vi "Stack_holderwise_total_bd_count_&_duration_3_for_stationwise.vi"(0 "Refnum in":T1, 1 "BREAKDOWN_STK_HOLD_ID":i32=1, 2 "condition":string="Where BREAKDOWN_DATE between '%s'and '%s' and BREAKDOWN_STK_HOLD_ID ='%d'  ", 5 "Form Date":timestamp, 7 "Array":string[](array[string]), 9 "To Date":timestamp, 11 "error in (no error)":errorcluster, 12 "STATION_ID_CID_TRIGGER":i32, 13 "Shift":string(combo), 14 "table":string[](array[string])=["STATION_1_LOG_HISTORY"]) -> (4 "Refnum out":T1, 6 "Count out":string[](array[string]), 10 "appended array":dbl[](array[numeric]), 15 "error out":errorcluster)   [LabVIEW 2017]
uses:
  <vilib>/addons/database/Connection.llb/Conn ObjectReference.ctl
  <vilib>/addons/database/NI_Database_API.lvlib
panel:
  out "Count out 2":string[](array[string])
  out "Table":string[][](array[string])
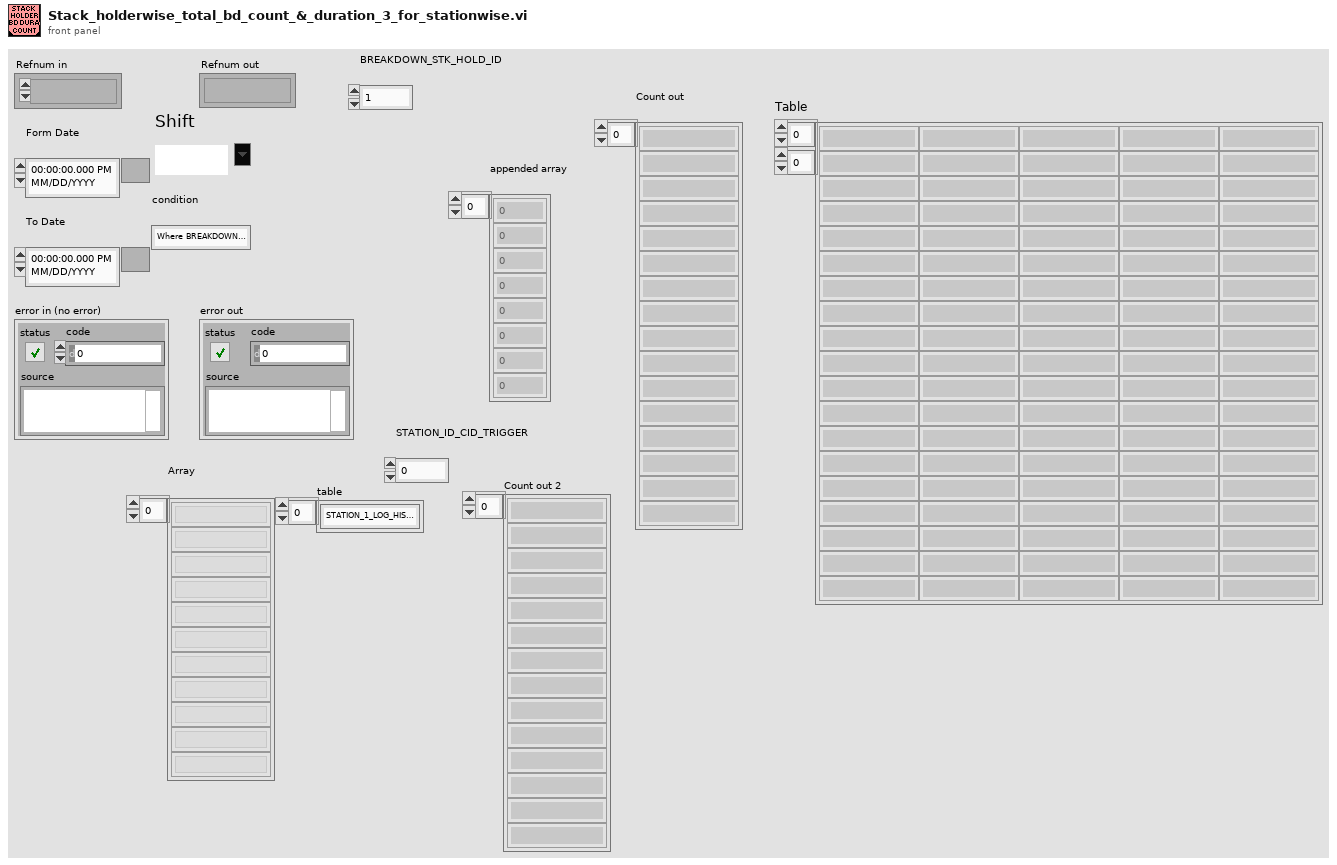
[diagram p1: front panel]
types:
  T1 = typedef "NI_Database_API.lvlib/Conn ObjectReference.ctl" = refnum<k1>
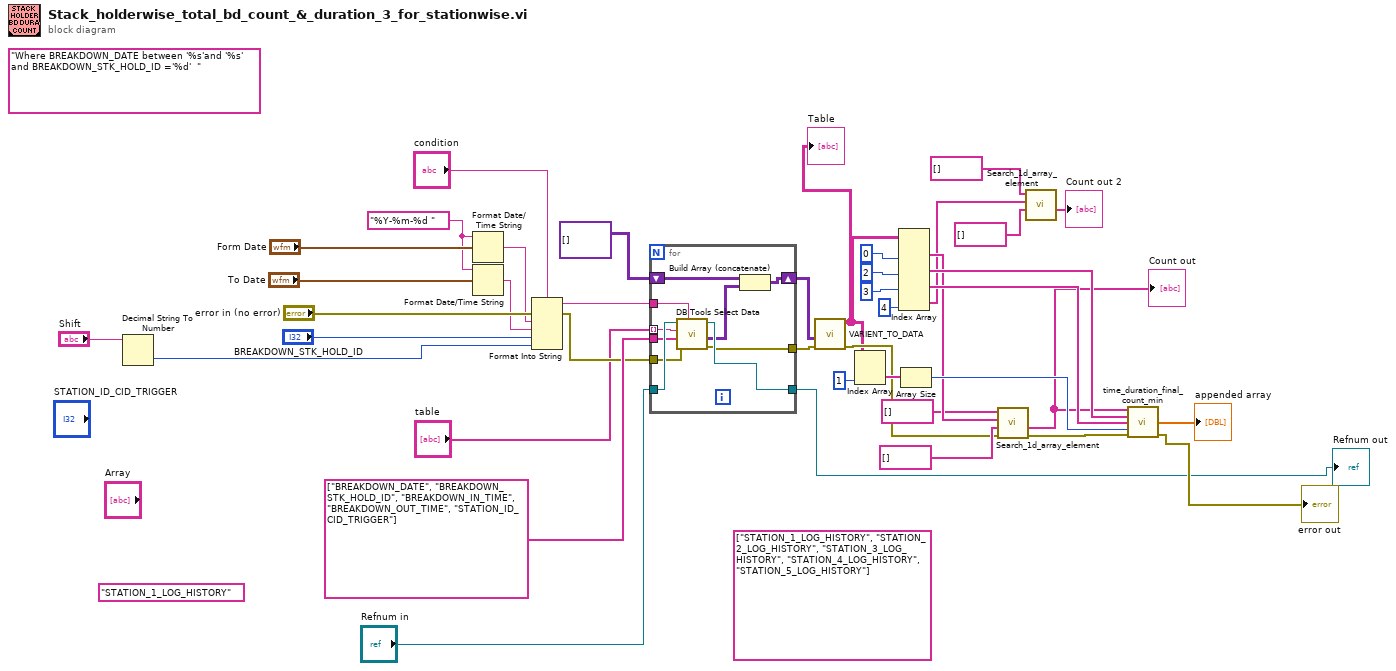
[diagram p0: block diagram]
diagram:
  (unwired) string[] ["STATION_1_LOG_HISTORY", "STATION_2_LOG_HISTORY", "STATION_3_LOG_HISTORY", "STATION_4_LOG_HISTORY", "STATION_5_LOG_HISTORY"]
  (unwired) "Where BREAKDOWN_DATE between '%s'and '%s' and BREAKDOWN_STK_HOLD_ID ='%d'  "
  (unwired) "STATION_1_LOG_HISTORY" ("table")
  w19 = "%Y-%m-%d " ("time format string (%c)")
  n1 = Decimal String To Number(string="Shift") -> (number=w12:i32)  [unwired: 2 in, 1 out]
  n2 = Format Date/Time String(time format string (%c)=w19, seconds (now)="Form Date") -> (date/time string=w22:string)  [unwired: 1 in]
  n3 = Format Date/Time String(time format string (%c)=w19, seconds (now)="To Date") -> (date/time string=w23:string)  [unwired: 1 in]
  n4 = Format Into String(format string="condition", error in="error in (no error)", w22, w23, "BREAKDOWN_STK_HOLD_ID", w12) -> (resulting string=w17:string, error out=w18:errorcluster)  [unwired: 1 in]
  n5 = for {
    tunnel: string[] ["BREAKDOWN_DATE", "BREAKDOWN_STK_HOLD_ID", "BREAKDOWN_IN_TIME", "BREAKDOWN_OUT_TIME", "STATION_ID_CID_TRIGGER"] -> [w47]
    tunnel: w17 -> [w48]
    tunnel: w18 -> [w49]
    tunnel: "table" -> [w46] mode=indexing
    tunnel: "Refnum in" -> [w50]
    tunnel: [w51] -> w26
    shift-right: [w44] -> w2
    shift-left: variant[][] [] ("data") -> [w45]
    tunnel: [w42] -> w4
    n6 = call <vilib>:"DB Tools Select Data.vi"("condition"=w48, "error in (no error)"=w49, "columns"=w47, "table"=w46, "connection reference"=w50) -> ("error out"=w42:errorcluster, "data"=w43:variant[][], "connection reference out"=w51:T1)  [unwired: 1 in]
    n7 = Build Array (concatenate)(w45, w43) -> (w44:variant[][])
  }
  "Refnum out" <- w26
  n8 = call "VARIENT_TO_DATA.vi"("data"=w2, "error in (no error)"=w4) -> ("Table"=w1:string[][], "error out"=w3:errorcluster)  [unwired: 7 in]
  "Table" <- w1
  n9 = Index Array(array=w1, index (col)=1 ("disabled index (col)")) -> (element=w33:string[])  [unwired: 1 in]
  n10 = Index Array(array=w1, index (col) #1=0 ("disabled index (col)"), index (col) #2=2 ("disabled index (col)"), index (col) #3=3 ("disabled index (col)"), index (col) #4=4 ("disabled index (col)")) -> (element #1=w35:string[], element #2=w37:string[], element #3=w38:string[], element #4=w10:string[])  [unwired: 4 in]
  n11 = Array Size(array=w33) -> (size(s)=w39:i32)
  n12 = call "Search_1d_array_element.vi"("error in (no error)"=w3, "Count in"=string[] [] ("Count"), "BD Date"=w35, "Elements Found in"=string[] [] ("Elements Found")) -> ("error out"=w36:errorcluster, "Count out"=w16:string[])  [unwired: 3 in, 1 out]
  "Count out" <- w16
  n13 = call "Search_1d_array_element.vi"("Count in"=string[] [] ("Count"), "BD Date"=w10, "Elements Found in"=string[] [] ("Elements Found")) -> ("Count out"=→"Count out 2":string[])  [unwired: 4 in, 2 out]
  n14 = call "time_duration_final_count_min.vi"("BD Count"=w16, "Intime"=w37, "OutTime"=w38, "bd array size"=w39, "error in (no error)"=w36) -> ("appended array"=→"appended array":dbl[], "error out"=→"error out":errorcluster)  [unwired: 7 in, 2 out]
